vi "GetHWI.vi"(8 "error in (no error)":errorcluster, 11 "Master Device in":refnum<class "Master Device.lvclass">) -> (0 "error out":errorcluster, 2 "Hardware Image":T2, 3 "Master Device out":refnum<class "Master Device.lvclass">)   [LabVIEW 2013, in "Master Device.lvclass"]
uses:
  Master Device.lvclass
  TypeDefs/RampInfo.ctl
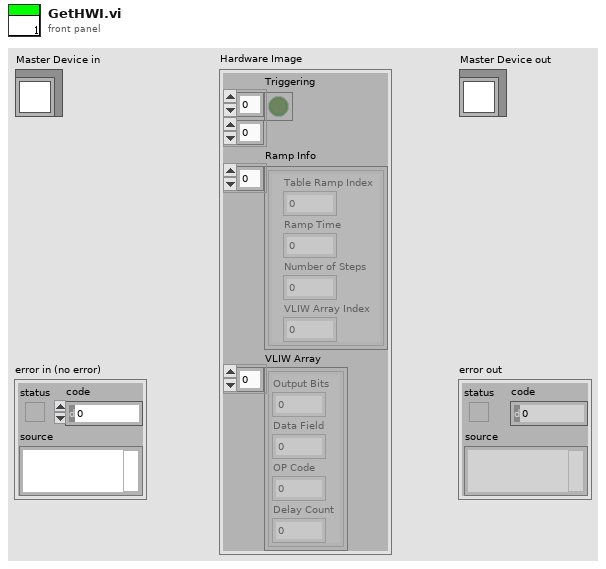
[diagram p1: front panel]
types:
  T1 = typedef "RampInfo.ctl" = cluster{"Table Ramp Index":i32, "Ramp Time":dbl, "Number of Steps":i32, "VLIW Array Index":i32}
  T2 = cluster{"Triggering":bool[][], "Ramp Info":T1[], "VLIW Array":cluster{"Output Bits":u32, "Data Field":u32, "OP Code":u8, "Delay Count":u64}[]}
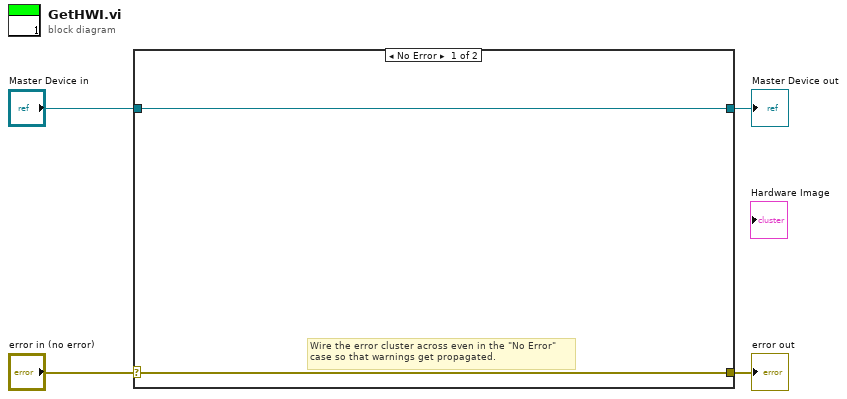
[diagram p0: block diagram]
diagram:
  n1 = case shown="No Error" "error in (no error)" {
    selector: "error in (no error)" -> [w5 w8]
    tunnel: [w5 w8] -> w3
    tunnel: [w6 w7] -> w1
    tunnel: "Master Device in" -> [w6 w7]
    frame No Error {
      # "Wire the error cluster across even in the \"No Error\"\ncase so that warnings get propagated."
    }
    frame Error {
    }
  }
  "error out" <- w3
  "Master Device out" <- w1
